vi "Find or make folder.vi"(8 "error in":errorcluster, 11 "Folder to find/make":path) -> (0 "error out":errorcluster, 2 "Made new":bool, 3 "created path":path)   [LabVIEW 2016]
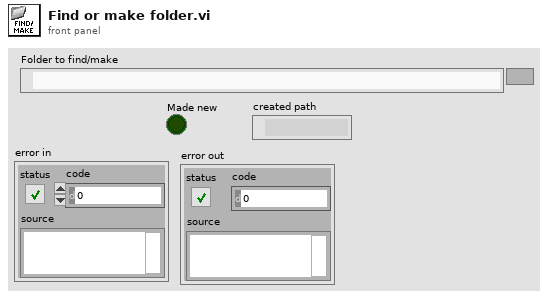
[diagram p1: front panel]
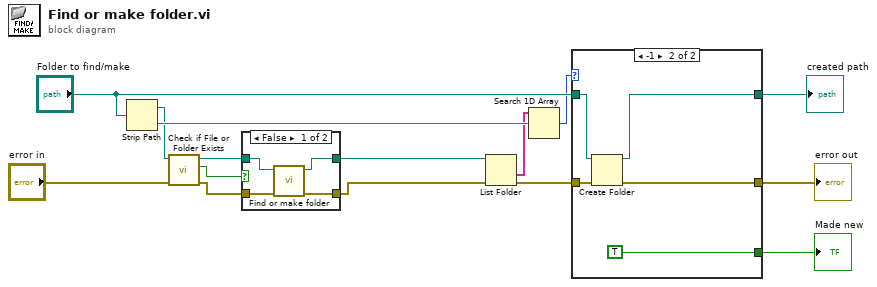
[diagram p0: block diagram]
diagram:
  n1 = Strip Path(path="Folder to find/make") -> (stripped path=w10:path, name=w15:string)
  n2 = call <vilib>:"Check if File or Folder Exists.vi"("error in (no error)"="error in", "path"=w10) -> ("error out"=w3:errorcluster, "file or folder exists?"=w4:bool, "dup path"=w5:path)  [unwired: 7 in]
  n3 = case shown="False" w4 {
    tunnel: w5 -> [w19 w21]
    tunnel: w3 -> [w18 w20]
    tunnel: [w17 w20] -> w2
    tunnel: [w16 w21] -> w1
    frame False {
      n4 = call "Find or make folder.vi"("error in"=w18, "Folder to find/make"=w19) -> ("error out"=w17:errorcluster, "created path"=w16:path)  [unwired: 7 in, 1 out]
    }
    frame True {
    }
  }
  n5 = List Folder(path=w1, error in=w2) -> (folder names=w8:string[], error out=w6:errorcluster)  [unwired: 2 in, 2 out]
  n6 = Search 1D Array(1D array=w8, element=w15) -> (index of element=w7:i32)  [unwired: 1 in]
  n7 = case shown="-1" w7 {
    tunnel: "Folder to find/make" -> [w23 w28]
    tunnel: [w23 w27] -> w11
    tunnel: w6 -> [w22 w26]
    tunnel: [w22 w25] -> w13
    tunnel: [_ TRUE] -> w12
    frame Default {
    }
    frame -1 {
      n8 = Create Folder(path (use dialog)=w28, error in=w26) -> (created path=w27:path, error out=w25:errorcluster)  [unwired: 1 in, 1 out]
    }
  }
  "error out" <- w13
  "Made new" <- w12
  "created path" <- w11
